vi "get status.vi"(8 "error in (no error)":errorcluster, 10 "status":u32, 11 "Relay Indetifier":i32=349111800) -> (0 "error out":errorcluster, 2 "status out":u32, 3 "Relay Indetifier Out":i32)   [LabVIEW 2022 SP3, in "usb_relay_device.lvlib"]
doc: "int EXPORT_API usb_relay_device_get_status(int hHandle, unsigned int *status);"
uses:
  usb_relay_device.lvlib
  usb_relay_device.dll
panel:
  out "function return":i32
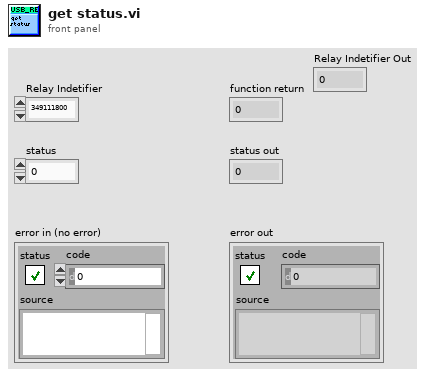
[diagram p1: front panel]
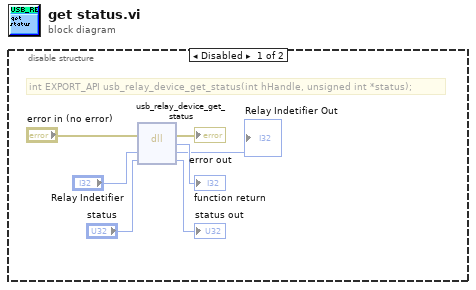
[diagram p0: block diagram]
diagram:
  n1 = disable-structure shown="Disabled" {
    frame Disabled {
      # "int EXPORT_API usb_relay_device_get_status(int hHandle, unsigned int *status);"
      n2 = dll-call lib="D:/LabVIEWSuite_64_OS/ScanningControl/Switch Modules/RiversideUSBRealy/usb_relay_device.*" fn="usb_relay_device_get_status"(error in="error in (no error)", "hHandle"="Relay Indetifier", "status"="status") -> (error out=→"error out":errorcluster, →"function return":i32, "hHandle"=→"Relay Indetifier Out":i32, "status"=→"status out":u32)  [unwired: 2 in, 1 out]
    }
    frame Enabled {
    }
  }
